vi "Slow Down.vi"(8 "error in (no error)":errorcluster, 11 "SwipeMenu in":refnum<class "SwipeMenu.lvclass">) -> (0 "error out":errorcluster, 3 "SwipeMenu out":refnum<class "SwipeMenu.lvclass">)   [LabVIEW 2019, in "SwipeMenu.lvclass"]
uses:
  SwipeMenu.lvclass
  SwipeMenu.lvclass/SwipeMenu.ctl
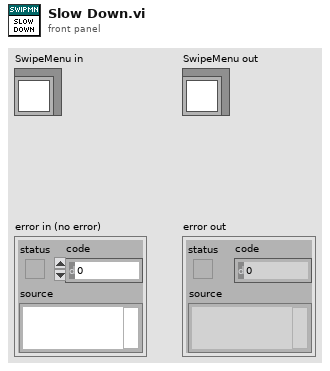
[diagram p1: front panel]
types:
  T1 = typedef "SwipeMenu.lvclass/State Data.ctl" = cluster{"State":enum16{"Idle", "Mouse Nav", "Slowdown", "Button Nav"}, "Timeout":i32, "Time":timestamp, "Position":i32, "Scroll Position":i16, "Rate":dbl, "Direction":enum16{"Left", "Right"}}
  T2 = enum16{"Idle", "Mouse Nav", "Slowdown", "Button Nav"}
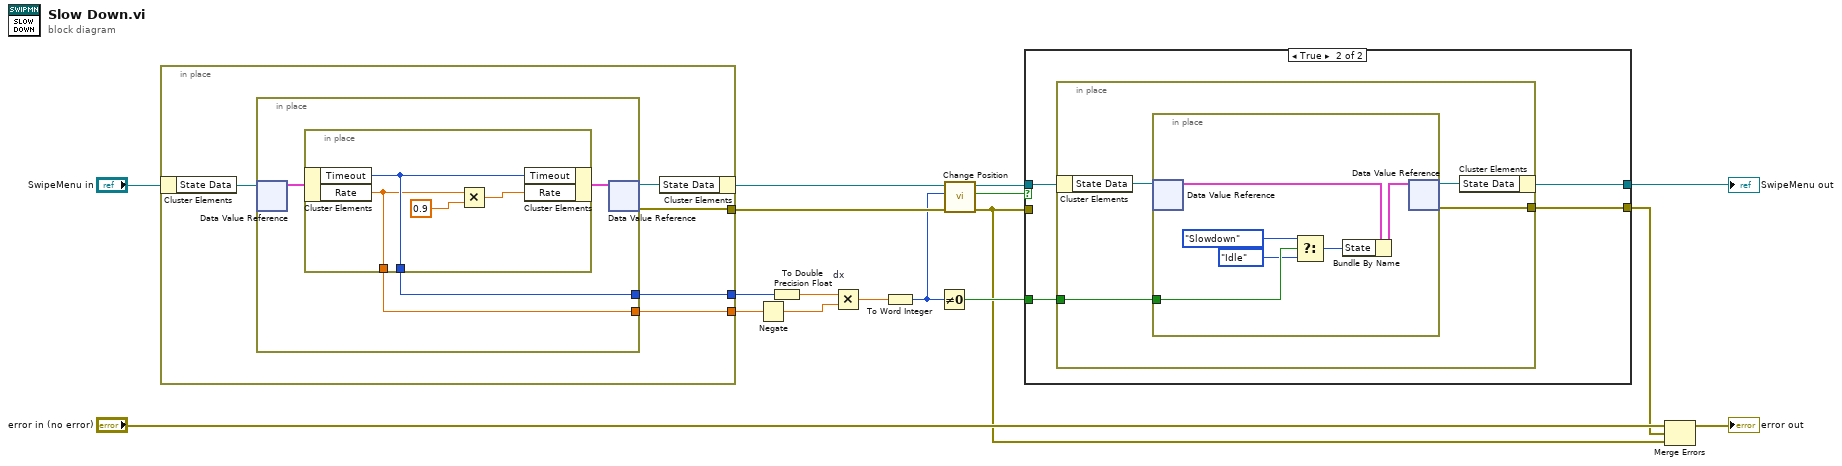
[diagram p0: block diagram]
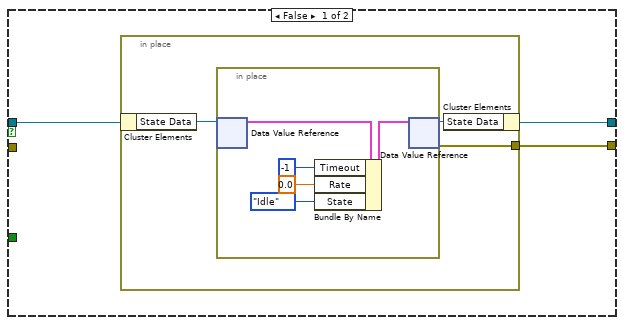
[diagram p2: hidden frame]
diagram:
  n1 = in-place {
    in-place-border: [w21] -> w17
    in-place-border: [w19] -> w9
    in-place-border: [w18] -> w4
    n2 = in-place-cluster #1("SwipeMenu in") -> ("State Data"=w22:refnum<data-value>)
    n3 = in-place {
      in-place-border: [w24] -> w21
      in-place-border: [w23] -> w19
      n4 = in-place-dvr #2(w22) -> (w26:T1)  [unwired: 1 out]
      n5 = in-place {
        in-place-border: [w28] -> w24
        in-place-border: [w27] -> w23
        n6 = in-place-cluster #3(w26) -> ("Timeout"=w28:i32, "Rate"=w27:dbl)
        n7 = Multiply(x=w27, y=0.9) -> (x*y=w29:dbl)
        n8 = in-place-cluster #3("Timeout"=w28, "Rate"=w29) -> (w25:T1)
      }
      n9 = in-place-dvr #2(w25) -> (w20:refnum<data-value>, w18:errorcluster)
    }
    n10 = in-place-cluster #1("State Data"=w20) -> (w6:refnum<class "SwipeMenu.lvclass">)
  }
  n11 = Negate(x=w9) -> (-x=w7:dbl)
  n12 = To Double Precision Float(number=w17) -> (double precision float=w15:dbl)
  n13 = Multiply "dx"(x=w15, y=w7) -> (x*y=w16:dbl)
  n14 = To Word Integer(number=w16) -> (16bit integer=w3:i16)
  n15 = Not Equal To 0?(x=w3) -> (x != 0?=w8:bool)
  n16 = call "Change Position.vi"("error in (no error)"=w4, "Change Position"=w3, "SwipeMenu in"=w6) -> ("error out"=w1:errorcluster, "In Range?"=w2:bool, "SwipeMenu out"=w5:refnum<class "SwipeMenu.lvclass">)  [unwired: 6 in]
  n17 = case shown="True" w2 {
    tunnel: w5 -> [w33 w45]
    tunnel: [w32 w44] -> w11
    tunnel: w1 -> [_ _]
    tunnel: [w31 w42] -> w12
    tunnel: w8 -> [_ w43]
    frame False {
      n18 = in-place {
        in-place-border: [w34] -> w31
        n19 = in-place-cluster #4(w33) -> ("State Data"=w36:refnum<data-value>)
        n20 = in-place {
          n21 = in-place-dvr #5(w36) -> (w39:T1)  [unwired: 1 out]
          n22 = Bundle By Name(cluster=w39, "Timeout"=-1, "Rate"=0.0, "State"=T2."Idle") -> (w38:T1)
          n23 = in-place-dvr #5(w38) -> (w35:refnum<data-value>, w34:errorcluster)
        }
        n24 = in-place-cluster #4("State Data"=w35) -> (w32:refnum<class "SwipeMenu.lvclass">)
      }
    }
    frame True {
      n25 = in-place {
        in-place-border: [w47] -> w42
        in-place-border: w43 -> [w46]
        n26 = in-place-cluster #6(w45) -> ("State Data"=w49:refnum<data-value>)
        n27 = in-place {
          in-place-border: w46 -> [w53]
          n28 = in-place-dvr #7(w49) -> (w55:T1)  [unwired: 1 out]
          n29 = Select(t=T2."Slowdown" ("State"), s=w53, f=T2."Idle" ("State")) -> (s? t:f=w50:T2)
          n30 = Bundle By Name(cluster=w55, "State"=w50) -> (w54:T1)
          n31 = in-place-dvr #7(w54) -> (w48:refnum<data-value>, w47:errorcluster)
        }
        n32 = in-place-cluster #6("State Data"=w48) -> (w44:refnum<class "SwipeMenu.lvclass">)
      }
    }
  }
  "SwipeMenu out" <- w11
  n33 = Merge Errors("error in (no error)", w12, w1) -> (→"error out":errorcluster)
